vi "Wash Timer.vi"(7 "Operation":enum16{"Init", "Read", "Pause"}(ring)) -> (2 "count":dbl)   [LabVIEW 2025]
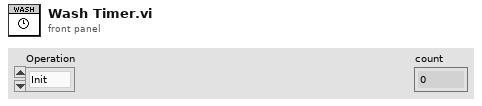
[diagram p1: front panel]
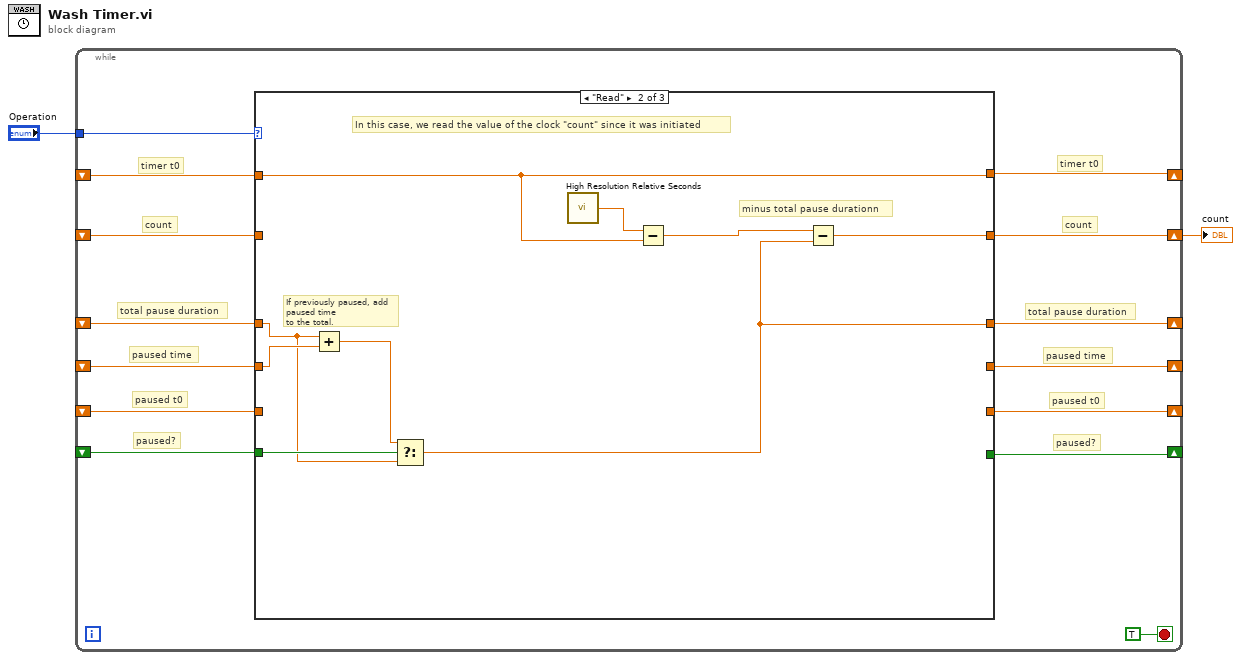
[diagram p0: block diagram]
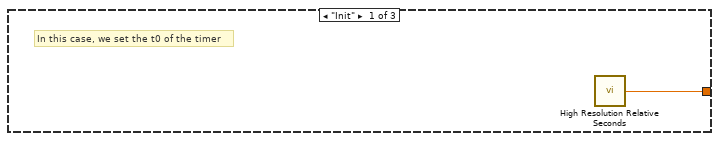
[diagram p2: hidden frame]
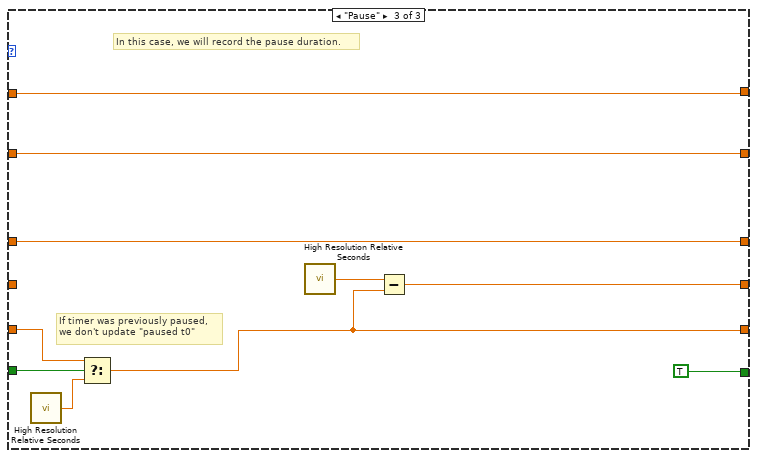
[diagram p3: hidden frame]
diagram:
  n1 = while {
    tunnel: "Operation" -> [w16]
    shift-right: [w15] -> _
    shift-left: _ -> [w14]
    shift-right: [w13] -> w1
    shift-left: _ -> [w12]
    shift-right: [w11] -> _
    shift-left: _ -> [w10]
    shift-right: [w9] -> _
    shift-left: _ -> [w8]
    shift-right: [w7] -> _
    shift-left: _ -> [w6]
    shift-right: [w5] -> _
    shift-left: _ -> [w4]
    stop <- TRUE stop-if-true
    # "total pause duration"
    # "total pause duration"
    # "paused time"
    # "paused time"
    # "paused t0"
    # "paused t0"
    # "paused?"
    # "paused?"
    # "count"
    # "count"
    # "timer t0"
    # "timer t0"
    n2 = case shown="\"Read\"" w16 {
      tunnel: [w17 w25 w36] -> w15
      tunnel: w14 -> [_ w25 w36]
      tunnel: [_ w19 w35] -> w13
      tunnel: w12 -> [_ _ w35]
      tunnel: [_ _ TRUE] -> w11
      tunnel: w10 -> [_ w24 w33]
      tunnel: [_ _ w29] -> w9
      tunnel: w8 -> [_ _ w31]
      tunnel: [_ _ w28] -> w7
      tunnel: w6 -> [_ w23 _]
      tunnel: [_ w18 w27] -> w5
      tunnel: w4 -> [_ w21 w27]
      frame "Init" {
        # "In this case, we set the t0 of the timer"
        n3 = call <vilib>:"High Resolution Relative Seconds.vi"() -> ("relative seconds"=w17:dbl)
      }
      frame "Read" {
        # "minus total pause durationn"
        # "If previously paused, add paused time\nto the total."
        # "In this case, we read the value of the clock \"count\" since it was initiated"
        n4 = Add(x=w21, y=w23) -> (x+y=w22:dbl)
        n5 = Select(t=w22, s=w24, f=w21) -> (s? t:f=w18:dbl)
        n6 = call <vilib>:"High Resolution Relative Seconds.vi"() -> ("relative seconds"=w26:dbl)
        n7 = Subtract(x=w26, y=w25) -> (x-y=w20:dbl)
        n8 = Subtract(x=w20, y=w18) -> (x-y=w19:dbl)
      }
      frame "Pause" {
        # "If timer was previously paused,\nwe don't update \"paused t0\""
        # "In this case, we will record the pause duration."
        n9 = call <vilib>:"High Resolution Relative Seconds.vi"() -> ("relative seconds"=w32:dbl)
        n10 = Select(t=w31, s=w33, f=w32) -> (s? t:f=w29:dbl)
        n11 = call <vilib>:"High Resolution Relative Seconds.vi"() -> ("relative seconds"=w30:dbl)
        n12 = Subtract(x=w30, y=w29) -> (x-y=w28:dbl)
      }
    }
  }
  "count" <- w1
